vi "laserShutDown.vi"(8 "error in (no error)":errorcluster, 9 "488prop":T1, 10 "553prop":T1, 11 "647prop":T1) -> (0 "error out":errorcluster)   [LabVIEW 2021]
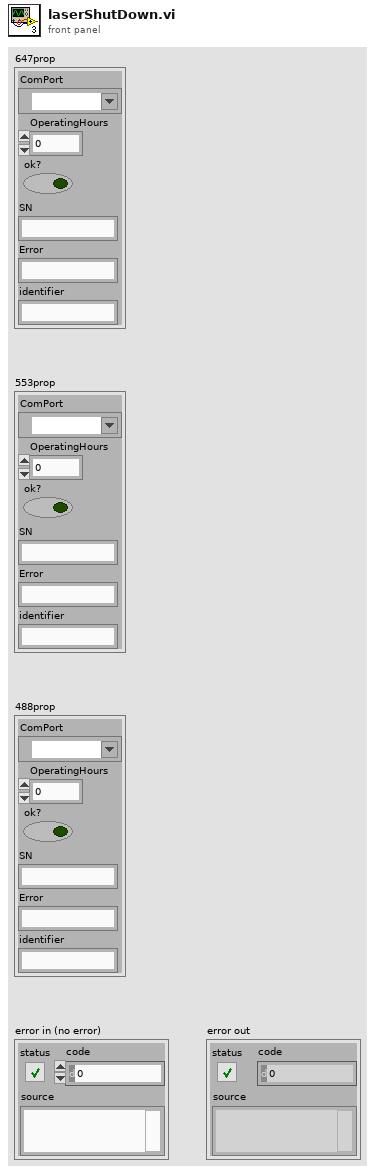
[diagram p1: front panel]
types:
  T1 = cluster{"ComPort":refnum<visa-resource-name>, "OperatingHours":dbl, "ok?":bool, "SN":string, "Error":string, "identifier":string}
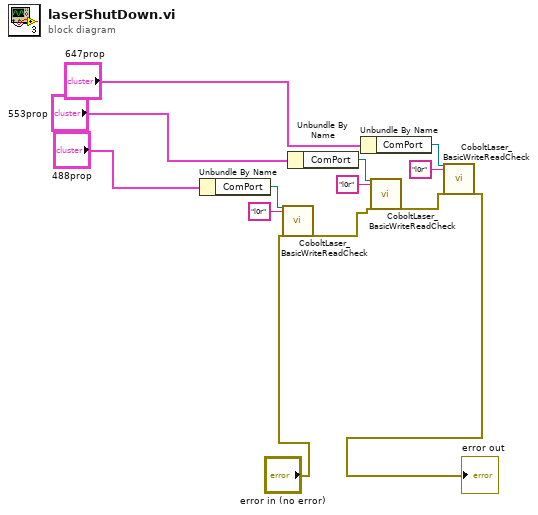
[diagram p0: block diagram]
diagram:
  n1 = Unbundle By Name("488prop") -> ("ComPort"=w1:refnum<visa-resource-name>)
  n2 = call "CoboltLaser_BasicWriteReadCheck.vi"("ComPort"=w1, "Command"="l0r", "error in (no error)"="error in (no error)") -> ("error out"=w9:errorcluster)  [unwired: 21 in, 3 out]
  n3 = Unbundle By Name("553prop") -> ("ComPort"=w6:refnum<visa-resource-name>)
  n4 = Unbundle By Name("647prop") -> ("ComPort"=w7:refnum<visa-resource-name>)
  n5 = call "CoboltLaser_BasicWriteReadCheck.vi"("ComPort"=w6, "Command"="l0r", "error in (no error)"=w9) -> ("error out"=w10:errorcluster)  [unwired: 21 in, 3 out]
  n6 = call "CoboltLaser_BasicWriteReadCheck.vi"("ComPort"=w7, "Command"="l0r", "error in (no error)"=w10) -> ("error out"=→"error out":errorcluster)  [unwired: 21 in, 3 out]
